vi "GetCurrentThread.vi"(4 "Manual thread":i64, 6 "Thread":T1, 8 "error in (no error)":errorcluster, 11 "Impersonate in":refnum<class "LogonUser.lvclass">) -> (0 "error out":errorcluster, 1 "thread id":i64, 3 "Impersonate out":refnum<class "LogonUser.lvclass">)   [LabVIEW 2018, in "LogonUser.lvclass"]
doc: "©2019\nWiebe Walstra\nwww.carya.nl"
uses:
  LogonUser.lvclass
  Threads.ctl
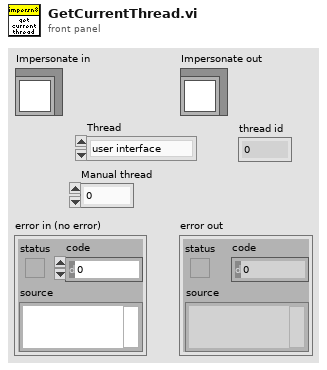
[diagram p1: front panel]
types:
  T1 = typedef "LogonUser.lvclass/Threads.ctl" = enum32{"user interface", "standard", "instrument i/o", "data acquisition", "other 1", "other 2", "same as caller", "manual"}
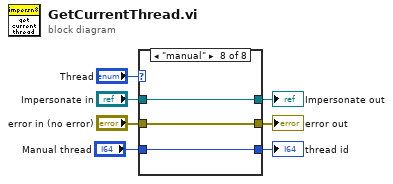
[diagram p0: block diagram]
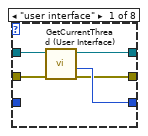
[diagram p2: hidden frame]
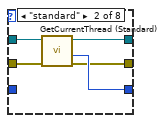
[diagram p3: hidden frame]
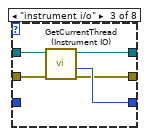
[diagram p4: hidden frame]
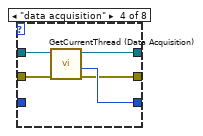
[diagram p5: hidden frame]
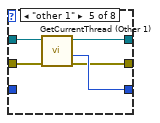
[diagram p6: hidden frame]
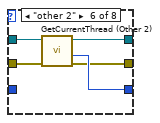
[diagram p7: hidden frame]
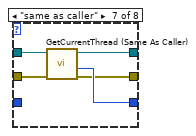
[diagram p8: hidden frame]
diagram:
  n1 = case shown="\"manual\"" "Thread" {
    tunnel: "error in (no error)" -> [w12 w17 w22 w27 w32 w37 w42 w44]
    tunnel: [w8 w13 w18 w23 w28 w33 w38 w44] -> w5
    tunnel: "Impersonate in" -> [w11 w16 w21 w26 w31 w36 w41 w45]
    tunnel: [w10 w15 w20 w25 w30 w35 w40 w45] -> w3
    tunnel: [w9 w14 w19 w24 w29 w34 w39 w43] -> w2
    tunnel: "Manual thread" -> [_ _ _ _ _ _ _ w43]
    frame "user interface" {
      n2 = call-dynamic "GetCurrentThread (User Interface).vi"("error in (no error)"=w12, "Impersonate in"=w11) -> ("error out"=w8:errorcluster, "thread id"=w9:i64, "Impersonate out"=w10:refnum<class "LogonUser.lvclass">)  [unwired: 7 in]
    }
    frame "standard" {
      n3 = call-dynamic "GetCurrentThread (Standard).vi"("error in (no error)"=w17, "Impersonate in"=w16) -> ("error out"=w13:errorcluster, "thread id"=w14:i64, "Impersonate out"=w15:refnum<class "LogonUser.lvclass">)  [unwired: 7 in]
    }
    frame "instrument i/o" {
      n4 = call-dynamic "GetCurrentThread (Instrument IO).vi"("error in (no error)"=w22, "Impersonate in"=w21) -> ("error out"=w18:errorcluster, "thread id"=w19:i64, "Impersonate out"=w20:refnum<class "LogonUser.lvclass">)  [unwired: 7 in]
    }
    frame "data acquisition" {
      n5 = call-dynamic "GetCurrentThread (Data Acquisition).vi"("error in (no error)"=w27, "Impersonate in"=w26) -> ("error out"=w23:errorcluster, "thread id"=w24:i64, "Impersonate out"=w25:refnum<class "LogonUser.lvclass">)  [unwired: 7 in]
    }
    frame "other 1" {
      n6 = call-dynamic "GetCurrentThread (Other 1).vi"("error in (no error)"=w32, "Impersonate in"=w31) -> ("error out"=w28:errorcluster, "thread id"=w29:i64, "Impersonate out"=w30:refnum<class "LogonUser.lvclass">)  [unwired: 7 in]
    }
    frame "other 2" {
      n7 = call-dynamic "GetCurrentThread (Other 2).vi"("error in (no error)"=w37, "Impersonate in"=w36) -> ("error out"=w33:errorcluster, "thread id"=w34:i64, "Impersonate out"=w35:refnum<class "LogonUser.lvclass">)  [unwired: 7 in]
    }
    frame "same as caller" {
      n8 = call-dynamic "GetCurrentThread (Same As Caller).vi"("error in (no error)"=w42, "Impersonate in"=w41) -> ("error out"=w38:errorcluster, "thread id"=w39:i64, "Impersonate out"=w40:refnum<class "LogonUser.lvclass">)  [unwired: 7 in]
    }
    frame "manual" {
    }
  }
  "error out" <- w5
  "Impersonate out" <- w3
  "thread id" <- w2
